vi "ShowAll.vi"(0 "reference in":refnum<class "CustomersBase.lvclass">, 5 "error in (no error)":errorcluster) -> (14 "reference out":refnum<class "CustomersBase.lvclass">, 19 "error out":errorcluster)   [LabVIEW 2020, in "CustomersBase.lvclass"]
uses:
  CustomersBase.lvclass
  DataObject_class/DataObject.lvclass
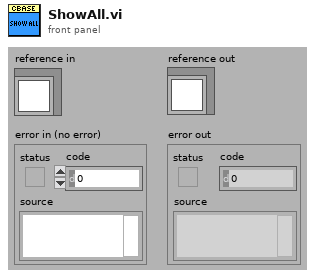
[diagram p1: front panel]
types:
  T1 = typedef "CustomersBase.lvclass/ObjectAttributes.ctl" = cluster{"_dataObject":refnum<class "DataObject.lvclass">, "Group":string}
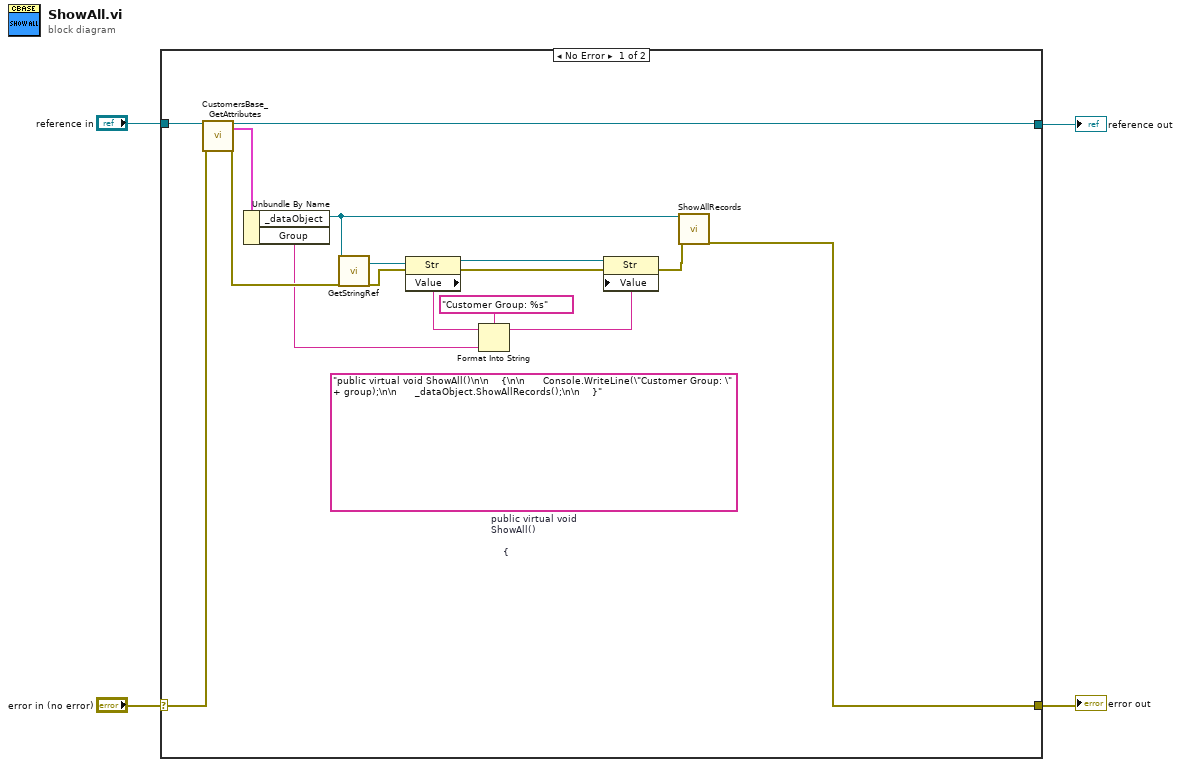
[diagram p0: block diagram]
diagram:
  n1 = case shown="No Error" "error in (no error)" {
    selector: "error in (no error)" -> [w19 w22]
    tunnel: [w16 w22] -> w3
    tunnel: [w17 w21] -> w1
    tunnel: "reference in" -> [w20 w21]
    frame No Error {
      (unwired) "public virtual void ShowAll()\n\n    {\n\n      Console.WriteLine(\"Customer Group: \" + group);\n\n      _dataObject.ShowAllRecords();\n\n    }"  # public virtual void ShowAll()      {        Console.WriteLine("Customer Group: " + group);        _dataObject.ShowAllRecords();      }
      n2 = call "CustomersBase_GetAttributes.vi"("reference in"=w20, "error in (no error)"=w19) -> ("reference out"=w17:refnum<class "CustomersBase.lvclass">, "Data"=w18:T1, "error out"=w11:errorcluster)  [unwired: 14 in, 1 out]
      n3 = Unbundle By Name(w18) -> ("_dataObject"=w10:refnum<class "DataObject.lvclass">, "Group"=w5:string)
      n4 = call-dynamic "GetStringRef.vi"("reference in"=w10, "error in (no error)"=w11) -> ("StringRef"=w15:refnum<vi>, "error out"=w12:errorcluster)  [unwired: 15 in, 1 out]
      n5 = property class="Str"(reference=w15, error in=w12) -> (reference out=w14:refnum<vi>, error out=w13:errorcluster, "Value"=w8:string)
      n6 = Format Into String(format string="Customer Group: %s", initial string=w8, w5) -> (resulting string=w7:string)  [unwired: 1 in, 1 out]
      n7 = property class="Str"(reference=w14, error in=w13, "Value"=w7) -> (error out=w9:errorcluster)  [unwired: 1 out]
      n8 = call-dynamic "ShowAllRecords.vi"("reference in"=w10, "error in (no error)"=w9) -> ("error out"=w16:errorcluster)  [unwired: 16 in, 1 out]
    }
    frame Error {
    }
  }
  "error out" <- w3
  "reference out" <- w1
